vi "Configure Timebase ZOOM.vi"(6 "Scale":T1(ring)=enum."5ms", 8 "error in (no error)":errorcluster, 9 "Offset (0)":dbl, 10 "Enable Zoom (F: Disable)":bool, 11 "VISA resource name":refnum<visa-resource-name>) -> (0 "error out":errorcluster, 3 "VISA resource name out":refnum<visa-resource-name>)   [LabVIEW 2015, in "ZhiYuan ZDS Series for TCP.lvlib"]
doc: "Configures the delay setting for timebase."
uses:
  ZhiYuan ZDS Series for TCP.lvlib
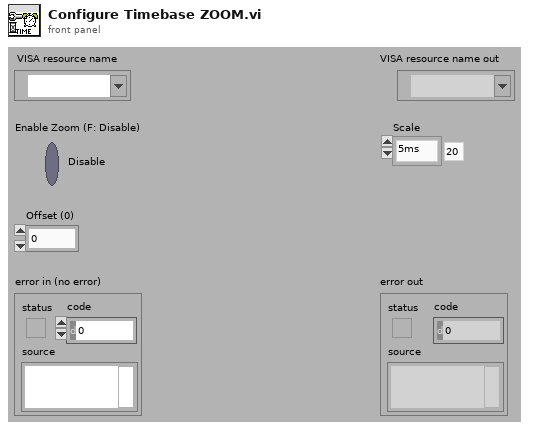
[diagram p1: front panel]
types:
  T1 = enum16{"1ns", "2ns", "5ns", "10ns", "20ns", "50ns", "100ns", "200ns", "500ns", "1us", "2us", "5us", "10us", "20us", "50us", "100us", "200us", "500us", "1ms", "2ms", "5ms", "10ms", "20ms", "50ms", "100ms", "200ms", "500ms", "1s", "2s", "5s", "10s", "20s", "50s", "100s"}
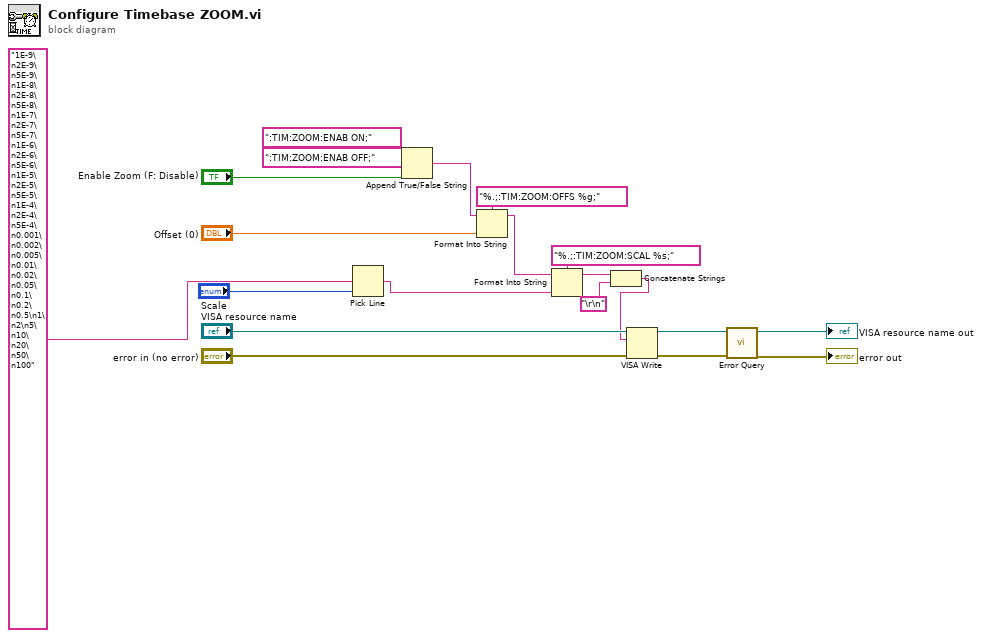
[diagram p0: block diagram]
diagram:
  n1 = Pick Line(multi-line string="1E-9\n2E-9\n5E-9\n1E-8\n2E-8\n5E-8\n1E-7\n2E-7\n5E-7\n1E-6\n2E-6\n5E-6\n1E-5\n2E-5\n5E-5\n1E-4\n2E-4\n5E-4\n0.001\n0.002\n0.005\n0.01\n0.02\n0.05\n0.1\n0.2\n0.5\n1\n2\n5\n10\n20\n50\n100", line index="Scale") -> (output string=w5:string)  [unwired: 1 in]
  n2 = Append True/False String(1:"Enable Zoom (F: Disable)", 2:":TIM:ZOOM:ENAB OFF;", 3:":TIM:ZOOM:ENAB ON;") -> (0:w17:string)  [unwired: 1 in]
  n3 = Format Into String(format string="%.;:TIM:ZOOM:OFFS %g;", initial string=w17, "Offset (0)") -> (resulting string=w14:string)  [unwired: 1 in, 1 out]
  n4 = Format Into String(format string="%.;:TIM:ZOOM:SCAL %s;", initial string=w14, w5) -> (resulting string=w4:string)  [unwired: 1 in, 1 out]
  n5 = Concatenate Strings(w4, "\r\n") -> (w2:string)
  n6 = VISA Write(VISA resource name="VISA resource name", write buffer=w2, error in (no error)="error in (no error)") -> (VISA resource name out=w10:refnum<visa-resource-name>, error out=w9:errorcluster)  [unwired: 1 out]
  n7 = call "Error Query.vi"("error in (no error)"=w9, "VISA resource name"=w10) -> ("error out"=→"error out":errorcluster, "VISA resource name out"=→"VISA resource name out":refnum<visa-resource-name>)  [unwired: 6 in, 2 out]
